vi "CheckCurrentMagnitude.vi"(9 "minimum current amps":dbl, 11 "current phasors":cdb[](array[numeric])) -> (1 "wiring info":string, 3 "> min current?":bool)   [LabVIEW 2017, in "McsaAnalysisLowRate.lvlib"]
uses:
  <vilib>/addons/InsightCM/Devices/Shared/Mcsa/McsaAnalysisLowRate/McsaAnalysisLowRate.lvlib
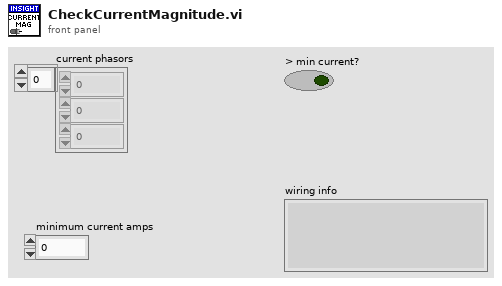
[diagram p1: front panel]
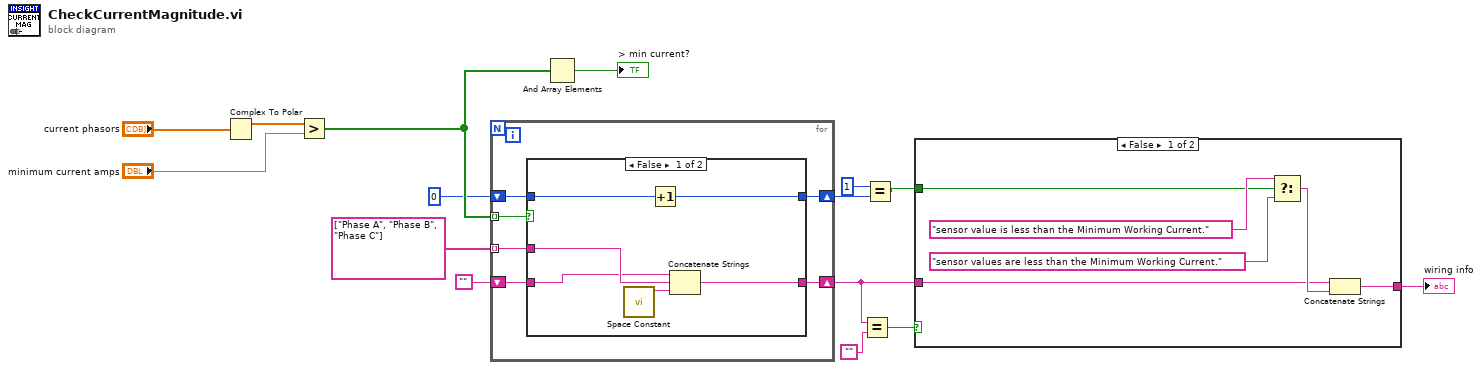
[diagram p0: block diagram]
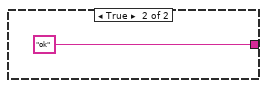
[diagram p2: hidden frame]
diagram:
  n1 = Complex To Polar(r * e^(i*theta)="current phasors") -> (r=w1:dbl[])  [unwired: 1 out]
  n2 = Greater?(x=w1, y="minimum current amps") -> (0:w11:bool[])
  n3 = for {
    tunnel: string[] ["Phase A", "Phase B", "Phase C"] -> [w19] mode=indexing
    shift-right: [w20] -> w8
    shift-left: "" -> [w21]
    tunnel: w11 -> [w18] mode=indexing
    shift-right: [w17] -> w5
    shift-left: 0 -> [w16]
    n4 = case shown="False" w18 {
      tunnel: w21 -> [w25 w29]
      tunnel: [w27 w29] -> w20
      tunnel: w19 -> [w26 _]
      tunnel: [w23 w28] -> w17
      tunnel: w16 -> [w24 w28]
      frame False {
        n5 = call <vilib>:"Space Constant.vi"() -> ("String"=w22:string)
        n6 = Increment(x=w24) -> (x+1=w23:i32)
        n7 = Concatenate Strings(w25, w26, w22) -> (w27:string)
      }
      frame True {
      }
    }
  }
  n8 = And Array Elements(Boolean array=w11) -> (logical AND=→"> min current?":bool)
  n9 = Equal?(x=w8, y="") -> (x = y?=w9:bool)
  n10 = Equal?(x=1, y=w5) -> (x = y?=w3:bool)
  n11 = case shown="False" w9 {
    tunnel: w8 -> [w32 _]
    tunnel: [w31 "ok"] -> w10
    tunnel: w3 -> [w30 _]
    frame False {
      n12 = Select(t="sensor value is less than the Minimum Working Current.", s=w30, f="sensor values are less than the Minimum Working Current.") -> (s? t:f=w34:string)
      n13 = Concatenate Strings(w32, w34) -> (w31:string)
    }
    frame True {
    }
  }
  "wiring info" <- w10
